vi "get_omega.vi"(2 "error in (no error)":errorcluster, 3 "M":dbl) -> (0 "error out":errorcluster, 1 "omega":dbl)   [LabVIEW 2021]
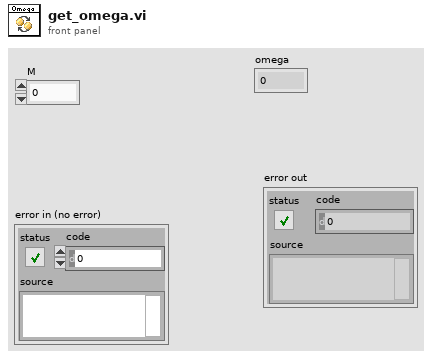
[diagram p1: front panel]
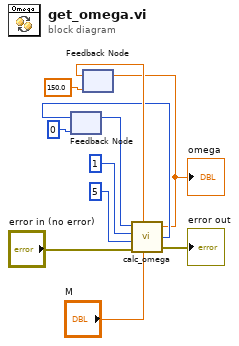
[diagram p0: block diagram]
diagram:
  n1 = feedback #1(i64 0 ("Nc")) -> (w8:i64)
  n2 = feedback #2(150.0 ("omega")) -> (w11:dbl)
  n3 = call "calc_omega.vi"("OldNc"=w8, "prev_omega"=w11, "MaxDeltaNc"=i64 1, "MaxNc"=i64 5, "M"="M", "error in (no error)"="error in (no error)") -> ("omega"=w5:dbl, "Nc"=w9:i64, "error out"=→"error out":errorcluster)
  "omega" <- w5
  n4 = feedback-in #1(w9) -> ()
  n5 = feedback-in #2(w5) -> ()
